vi "Image Filter 8x8 (SubVI).vi"(0 "Data In":u8, 1 "Data Valid?":bool) -> (14 "Data Out":u64, 15 "Output Valid?":bool)   [LabVIEW 2015]
doc: "Filters input image and remove objects that are smaller than 128 x 128 pixels in size."
uses:
  <vilib>/rvi/Emulation/niFpgaSctlEmulationGetInTimedLoop.vi
  <vilib>/Utility/error.llb/Clear Errors.vi
  <vilib>/rvi/DataTransferAndStorage/Container/Common/niFpgaContainerGetUniqueNameForEmu.vi
  <vilib>/rvi/DataTransferAndStorage/Container/Common/niFpgaContainerSetEmuInfo.vi
  <vilib>/rvi/eio/common/nirviEmuReportErrorAndStop.vi
  <vilib>/rvi/Emulation/niFpgaEmulationIsFPGAContextNoSignature.vi
  <vilib>/rvi/errors/niFpgaSetErrorForExecOnDevCompSimple.vi
  <vilib>/rvi/FIFO/Fifo_Resource/nirvififoEmulationSetSize.vi
  <vilib>/rvi/FIFO/Fifo_Resource/nirviFifoEmulationQueueMgr.vi
  <instcachedir>/0/nirviFifoEmulationQueueMgr_E5CAEC123FF24DC58D834DCA3CDAA9B5.lvgen/nirviFifoEmulationQueueMgr_E5CAEC123FF24DC58D834DCA3CDAA9B5_001.vi
  <vilib>/rvi/FIFO/Fifo_Resource/nirvififoEmulationCreateLock.vi
  <vilib>/rvi/Emulation/niFpgaProcessEmulError.vi
  <vilib>/rvi/FIFO/Fifo_Resource/nirvififoEmulationObtainLock.vi
  <vilib>/rvi/FIFO/Fifo_Resource/nirvififoEmulationReleaseLock.vi
  <vilib>/rvi/occurrence/nirviWaitOnOccurrenceBase.vi
  <vilib>/rvi/errors/nirviReportUnexpectedCaseInternalError.vi
  <vilib>/rvi/errors/nirviReportUnexpectedCaseInternalError (U32).vi
  <vilib>/rvi/FIFO/Fifo_Resource/nirvififoEmulationDetermineInputValidOut.vi
  <instcachedir>/0/nirviFifoEmulationQueueMgr_E5CAEC123FF24DC58D834DCA3CDAA9B5.lvgen/nirviFifoEmulationQueueMgr_E5CAEC123FF24DC58D834DCA3CDAA9B5_002.vi
  <vilib>/rvi/LocalResourceManager/LocalResourceManager.xnode
  <vilib>/rvi/DataTransferAndStorage/Container/XNode/niFpgaContainer.xnode
  <vilib>/rvi/FIFO/Fifo_Resource/nirvififoEmulationRead.vi
  <vilib>/rvi/FIFO/Fifo_Resource/nirvififoEmulationWrite.vi
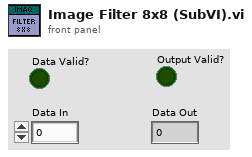
[diagram p1: front panel]
types:
  T1 = cluster{"Boolean array[0]":bool, "Boolean array[1]":bool, "Boolean array[2]":bool, "Boolean array[3]":bool, "Boolean array[4]":bool, "Boolean array[5]":bool, "Boolean array[6]":bool, "Boolean array[7]":bool}
  T2 = cluster{"Boolean array[0]":i16, "Boolean array[1]":i16, "Boolean array[2]":i16, "Boolean array[3]":i16, "Boolean array[4]":i16, "Boolean array[5]":i16, "Boolean array[6]":i16, "Boolean array[7]":i16}
  T3 = cluster{"Numeric Control":u8, "Numeric Control":u8, "Numeric Control":u8, "Numeric Control":u8, "Numeric Control":u8, "Numeric Control":u8, "Numeric Control":u8, "Numeric Control":u8}
  T4 = cluster{"Pixel 1":u8, "Pixel 2":u8, "Pixel 3":u8, "Pixel 4":u8, "Pixel 5":u8, "Pixel 6":u8, "Pixel 7":u8, "Pixel 8":u8}
  T5 = cluster{"Pixel 1":bool, "Pixel 2":bool, "Pixel 3":bool, "Pixel 4":bool, "Pixel 5":bool, "Pixel 6":bool, "Pixel 7":bool, "Pixel 8":bool}
  T6 = cluster{"Pixel 1":i16, "Pixel 2":i16, "Pixel 3":i16, "Pixel 4":i16, "Pixel 5":i16, "Pixel 6":i16, "Pixel 7":i16, "Pixel 8":i16}
  T7 = cluster{"Boolean array[0]":u8, "Boolean array[1]":u8, "Boolean array[2]":u8, "Boolean array[3]":u8, "Boolean array[4]":u8, "Boolean array[5]":u8, "Boolean array[6]":u8, "Boolean array[7]":u8}
  T8 = cluster{"t":u8, "t":u8, "t":u8, "t":u8, "t":u8, "t":u8, "t":u8, "t":u8}
  T9 = cluster{"t":bool, "t":bool, "t":bool, "t":bool, "t":bool, "t":bool, "t":bool, "t":bool}
  T10 = cluster{bool, bool, bool, bool, bool, bool, bool, bool}
  T11 = cluster{"[0]":u8, "[1]":u8, "[2]":u8, "[3]":u8, "[4]":u8, "[5]":u8, "[6]":u8, "[7]":u8}
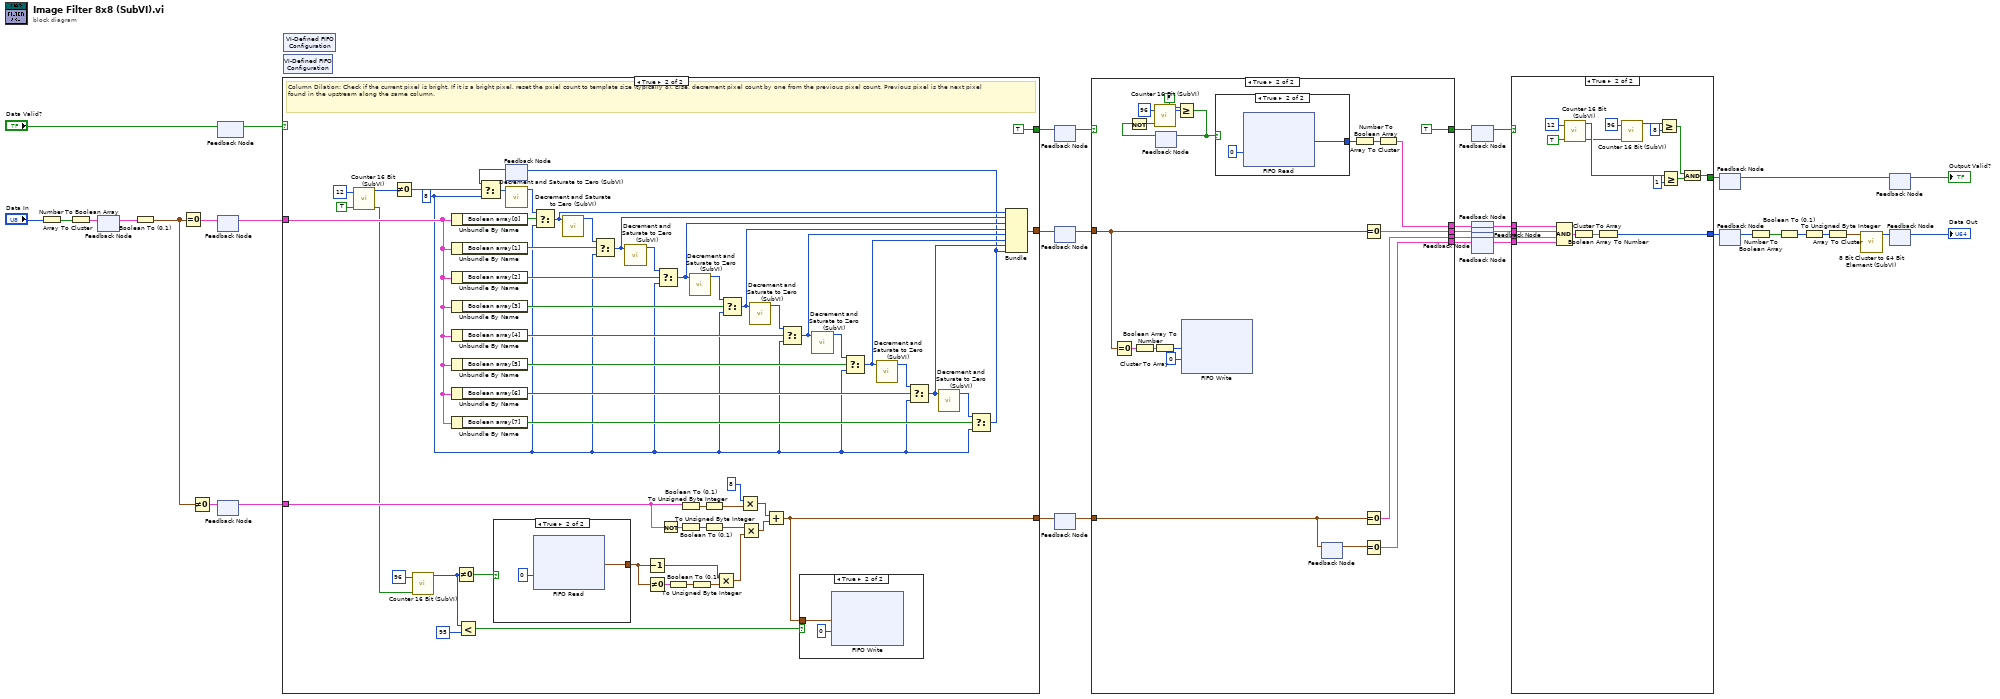
[diagram p0: block diagram]
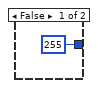
[diagram p4: hidden frame]
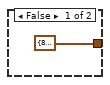
[diagram p7: hidden frame]
diagram:
  n1 = Number To Boolean Array(number="Data In") -> (Boolean array=w12:bool[])
  n2 = Array To Cluster(array=w12) -> (cluster=w11:T1)
  n3 = feedback-in #1(w11) -> ()
  n4 = feedback #1() -> (w14:T1)  [unwired: 1 in]
  n5 = Boolean To (0,1)(Boolean=w14) -> (0, 1=w10:T2)
  n6 = Equal To 0?(x=w10) -> (x = 0?=w31:T1)
  n7 = Not Equal To 0?(x=w10) -> (x != 0?=w9:T1)
  n8 = feedback-in #2("Data Valid?") -> ()
  n9 = feedback #2() -> (w28:bool)  [unwired: 1 in]
  n10 = feedback-in #3(w31) -> ()
  n11 = feedback #3() -> (w29:T1)  [unwired: 1 in]
  n12 = feedback-in #4(w9) -> ()
  n13 = feedback #4() -> (w30:T1)  [unwired: 1 in]
  n14 = case shown="True" w28 {
    tunnel: [_ w92] -> w37
    tunnel: [_ TRUE] -> w36
    tunnel: [_ w49] -> w38
    tunnel: w29 -> [_ w48]
    tunnel: w30 -> [_ w47]
    frame False {
    }
    frame True {
      w43 = u8 8 ("t")
      # "Column Dilation: Check if the current pixel is bright. If it is a bright pixel, reset the pxiel count to template size (typically 8). Else, decrement pixel count by one from the previous pixel count. Previous pixel is the next pixel found in the upstream along the same column."
      n15 = call "Counter 16 Bit (SubVI).vi"("Max. Count"=u16 12, "Enable"=TRUE) -> ("Count"=w44:u16, "Count End?"=w45:bool)  [unwired: 11 in, 1 out]
      n16 = Not Equal To 0?(x=w44) -> (x != 0?=w46:bool)
      n17 = call "Counter 16 Bit (SubVI).vi"("Max. Count"=u16 96, "Enable"=w45) -> ("Count"=w41:u16)  [unwired: 11 in, 2 out]
      n18 = Unbundle By Name(w48) -> ("Boolean array[0]"=w88:bool)
      n19 = Unbundle By Name(w48) -> ("Boolean array[1]"=w87:bool)
      n20 = Unbundle By Name(w48) -> ("Boolean array[2]"=w84:bool)
      n21 = Unbundle By Name(w48) -> ("Boolean array[3]"=w79:bool)
      n22 = Unbundle By Name(w48) -> ("Boolean array[4]"=w80:bool)
      n23 = Unbundle By Name(w48) -> ("Boolean array[5]"=w83:bool)
      n24 = Unbundle By Name(w48) -> ("Boolean array[6]"=w77:bool)
      n25 = Unbundle By Name(w48) -> ("Boolean array[7]"=w74:bool)
      n26 = Not Equal To 0?(x=w41) -> (x != 0?=w65:bool)
      n27 = Less?(x=w41, y=u16 95) -> (x < y?=w59:bool)
      n28 = case shown="True" w65 {
        tunnel: [T3 {"Numeric Control"=8, "Numeric Control"=8, "Numeric Control"=8, "Numeric Control"=8, "Numeric Control"=8, "Numeric Control"=8, "Numeric Control"=8, "Numeric Control"=8} ("Cluster") w99] -> w60
        frame False {
        }
        frame True {
          n29 = xnode ("FIFO Read")("Timeout"=0) -> ("Element"=w99:T4)  [unwired: 1 in, 2 out]
        }
      }
      n30 = feedback #5() -> (w91:u8)  [unwired: 1 in]
      n31 = Select(t=w91, s=w46, f=w43) -> (s? t:f=w90:u8)
      n32 = call "Decrement and Saturate to Zero (SubVI).vi"("Data In"=w90) -> ("Data Out"=w89:u8)  [unwired: 10 in]
      n33 = Select(t=w89, s=w88, f=w43) -> (s? t:f=w73:u8)
      n34 = call "Decrement and Saturate to Zero (SubVI).vi"("Data In"=w73) -> ("Data Out"=w86:u8)  [unwired: 10 in]
      n35 = Select(t=w86, s=w87, f=w43) -> (s? t:f=w72:u8)
      n36 = call "Decrement and Saturate to Zero (SubVI).vi"("Data In"=w72) -> ("Data Out"=w85:u8)  [unwired: 10 in]
      n37 = Decrement(x=w60) -> (x-1=w64:T4)
      n38 = Not Equal To 0?(x=w60) -> (x != 0?=w61:T5)
      n39 = Select(t=w85, s=w84, f=w43) -> (s? t:f=w71:u8)
      n40 = Not(x=w47) -> (.not. x?=w55:T1)
      n41 = Boolean To (0,1)(Boolean=w61) -> (0, 1=w62:T6)
      n42 = Boolean To (0,1)(Boolean=w47) -> (0, 1=w57:T2)
      n43 = Boolean To (0,1)(Boolean=w55) -> (0, 1=w53:T2)
      n44 = call "Decrement and Saturate to Zero (SubVI).vi"("Data In"=w71) -> ("Data Out"=w78:u8)  [unwired: 10 in]
      n45 = To Unsigned Byte Integer(number=w62) -> (unsigned 8bit integer=w63:T4)
      n46 = To Unsigned Byte Integer(number=w57) -> (unsigned 8bit integer=w58:T7)
      n47 = To Unsigned Byte Integer(number=w53) -> (unsigned 8bit integer=w54:T7)
      n48 = Multiply(x=w64, y=w63) -> (x*y=w52:T4)
      n49 = Select(t=w78, s=w79, f=w43) -> (s? t:f=w70:u8)
      n50 = Multiply(x=u8 8 ("unsigned 8bit integer"), y=w58) -> (x*y=w51:T7)
      n51 = Multiply(x=w54, y=w52) -> (x*y=w50:cluster{u8, u8, u8, u8, u8, u8, u8, u8})
      n52 = call "Decrement and Saturate to Zero (SubVI).vi"("Data In"=w70) -> ("Data Out"=w81:u8)  [unwired: 10 in]
      n53 = Add(x=w51, y=w50) -> (x+y=w49:cluster{u8, u8, u8, u8, u8, u8, u8, u8})
      n54 = Select(t=w81, s=w80, f=w43) -> (s? t:f=w69:u8)
      n55 = case shown="True" w59 {
        tunnel: w49 -> [_ w96]
        frame False {
        }
        frame True {
          n56 = xnode ("FIFO Write")("Element"=w96, "Timeout"=0) -> ()  [unwired: 1 in, 2 out]
        }
      }
      n57 = call "Decrement and Saturate to Zero (SubVI).vi"("Data In"=w69) -> ("Data Out"=w82:u8)  [unwired: 10 in]
      n58 = Select(t=w82, s=w83, f=w43) -> (s? t:f=w68:u8)
      n59 = call "Decrement and Saturate to Zero (SubVI).vi"("Data In"=w68) -> ("Data Out"=w76:u8)  [unwired: 10 in]
      n60 = Select(t=w76, s=w77, f=w43) -> (s? t:f=w67:u8)
      n61 = call "Decrement and Saturate to Zero (SubVI).vi"("Data In"=w67) -> ("Data Out"=w75:u8)  [unwired: 10 in]
      n62 = Select(t=w75, s=w74, f=w43) -> (s? t:f=w66:u8)
      n63 = feedback-in #5(w66) -> ()
      n64 = Bundle("t"=w73, "t"=w72, "t"=w71, "t"=w70, "t"=w69, "t"=w68, "t"=w67, "t"=w66) -> (w92:T8)  [unwired: 1 in]
    }
  }
  n65 = xnode "VI-Defined FIFO Configuration"() -> ()  [unwired: 1 out]
  n66 = xnode "VI-Defined FIFO Configuration"() -> ()  [unwired: 1 out]
  n67 = feedback-in #6(w36) -> ()
  n68 = feedback #6() -> (w35:bool)  [unwired: 1 in]
  n69 = feedback-in #7(w37) -> ()
  n70 = feedback #7() -> (w34:T8)  [unwired: 1 in]
  n71 = feedback-in #8(w38) -> ()
  n72 = feedback #8() -> (w33:T4)  [unwired: 1 in]
  n73 = case shown="True" w35 {
    tunnel: w34 -> [_ w114]
    tunnel: w33 -> [_ w119]
    tunnel: [_ TRUE] -> w26
    tunnel: [_ w106] -> w24
    tunnel: [_ w105] -> w23
    tunnel: [_ w104] -> w22
    tunnel: [_ w103] -> w21
    frame False {
    }
    frame True {
      w102 = u16 96 ("Max. Count")
      n74 = Equal To 0?(x=w114) -> (x = 0?=w116:T9)
      n75 = Cluster To Array(cluster=w116) -> (array=w115:bool[])
      n76 = Boolean Array To Number(Boolean array=w115) -> (number=w110:u8)
      n77 = feedback #9() -> (w112:bool)  [unwired: 1 in]
      n78 = Not(x=w112) -> (.not. x?=w107:bool)
      n79 = call "Counter 16 Bit (SubVI).vi"("Max. Count"=w102, "Auto RESET"=FALSE, "Enable"=w107) -> ("Count"=w101:u16)  [unwired: 10 in, 2 out]
      n80 = Greater Or Equal?(x=w101, y=w102) -> (x >= y?=w108:bool)
      n81 = feedback-in #9(w108) -> ()
      n82 = xnode ("FIFO Write")("Element"=w110, "Timeout"=0) -> ()  [unwired: 1 in, 2 out]
      n83 = case shown="True" w108 {
        tunnel: [u8 255 ("Element") w121] -> w109
        frame False {
        }
        frame True {
          n84 = xnode ("FIFO Read")("Timeout"=0) -> ("Element"=w121:u8)  [unwired: 1 in, 2 out]
        }
      }
      n85 = feedback #10() -> (w118:T4)  [unwired: 1 in]
      n86 = feedback-in #10(w119) -> ()
      n87 = Number To Boolean Array(number=w109) -> (Boolean array=w113:bool[])
      n88 = Equal To 0?(x=w114) -> (x = 0?=w105:T9)
      n89 = Equal To 0?(x=w119) -> (x = 0?=w104:T5)
      n90 = Equal To 0?(x=w118) -> (x = 0?=w103:T5)
      n91 = Array To Cluster(array=w113) -> (cluster=w106:T1)
    }
  }
  n92 = feedback-in #11(w26) -> ()
  n93 = feedback #11() -> (w16:bool)  [unwired: 1 in]
  n94 = feedback-in #12(w24) -> ()
  n95 = feedback #12() -> (w17:T1)  [unwired: 1 in]
  n96 = feedback-in #13(w23) -> ()
  n97 = feedback #13() -> (w18:T9)  [unwired: 1 in]
  n98 = feedback-in #14(w22) -> ()
  n99 = feedback #14() -> (w19:T5)  [unwired: 1 in]
  n100 = feedback-in #15(w21) -> ()
  n101 = feedback #15() -> (w20:T5)  [unwired: 1 in]
  n102 = case shown="True" w16 {
    tunnel: [_ w128] -> w27
    tunnel: [_ w131] -> w25
    tunnel: w17 -> [_ w140]
    tunnel: w18 -> [_ w139]
    tunnel: w19 -> [_ w138]
    tunnel: w20 -> [_ w137]
    frame False {
    }
    frame True {
      n103 = Compound Arithmetic op=AND(w140, w139, w138, w137) -> (w130:T10)
      n104 = call "Counter 16 Bit (SubVI).vi"("Max. Count"=u16 12, "Enable"=TRUE) -> ("Count"=w127:u16, "Count End?"=w126:bool)  [unwired: 11 in, 1 out]
      n105 = Cluster To Array(cluster=w130) -> (array=w129:bool[])
      n106 = Boolean Array To Number(Boolean array=w129) -> (number=w128:u8)
      n107 = call "Counter 16 Bit (SubVI).vi"("Max. Count"=u16 96, "Enable"=w126) -> ("Count"=w125:u16)  [unwired: 11 in, 2 out]
      n108 = Greater Or Equal?(x=w125, y=u16 8 ("t")) -> (x >= y?=w133:bool)
      n109 = Greater Or Equal?(x=w127, y=u16 1 ("t")) -> (x >= y?=w132:bool)
      n110 = And(x=w133, y=w132) -> (x .and. y?=w131:bool)
    }
  }
  n111 = feedback-in #16(w25) -> ()
  n112 = feedback #16() -> (w15:bool)  [unwired: 1 in]
  n113 = feedback-in #17(w27) -> ()
  n114 = feedback #17() -> (w8:u8)  [unwired: 1 in]
  n115 = Number To Boolean Array(number=w8) -> (Boolean array=w6:bool[])
  n116 = Boolean To (0,1)(Boolean=w6) -> (0, 1=w5:i16[])
  n117 = To Unsigned Byte Integer(number=w5) -> (unsigned 8bit integer=w4:u8[])
  n118 = Array To Cluster(array=w4) -> (cluster=w3:T11)
  n119 = call "8 Bit Cluster to 64 Bit Element (SubVI).vi"("Pixel Cluster"=w3) -> ("Pixel Data (64-Bit)"=w7:u64)  [unwired: 10 in]
  n120 = feedback-in #18(w15) -> ()
  n121 = feedback #18() -> (→"Output Valid?":bool)  [unwired: 1 in]
  n122 = feedback-in #19(w7) -> ()
  n123 = feedback #19() -> (→"Data Out":u64)  [unwired: 1 in]
